vi "Grover Search.vi"   [LabVIEW 2020]
uses:
  QuSim/QuVI_Wire (initial).vi
  QuSim/QuVI_Wire (added).vi
  Gates/Polymorphs/Pauli-X_s.vi
  Gates/Polymorphs/vAControl_e.vi
  Gates/Polymorphs/vAControl_m.vi
  Gates/Polymorphs/Pauli-Z_t.vi
  Gates/Polymorphs/vControl_e.vi
  Gates/Polymorphs/vControl_m.vi
  Analysis/Inspect VIs/Probability Bar.vi
  QuSim/QuWire/QuWire.lvclass
panel:
  # "Grover Search Example"
  # "*Open the block diagram for the circuit view (Ctrl+E)"
  # "Performs Grover's Search algorithm to find a marked item in a 4-qubit space (N=16).\n\nThis VI demonstrates amplitude amplification. It uses a 'For Loop' to iterate the Oracle and Diffusion operators approx. 3 times (optimal for N=16). A 'Case Structure' inside allows you to dynamically select which state (e.g., |1010>) is marked by the Oracle. Watch the probability of the target state rise to >96%."
types:
  T1 = enum16{"0000", "0001", "0010", "0011", "0100", "0101", "0110", "0111", "1000", "1001", "1010", "1011", "1100", "1101", "1110", "1111"}
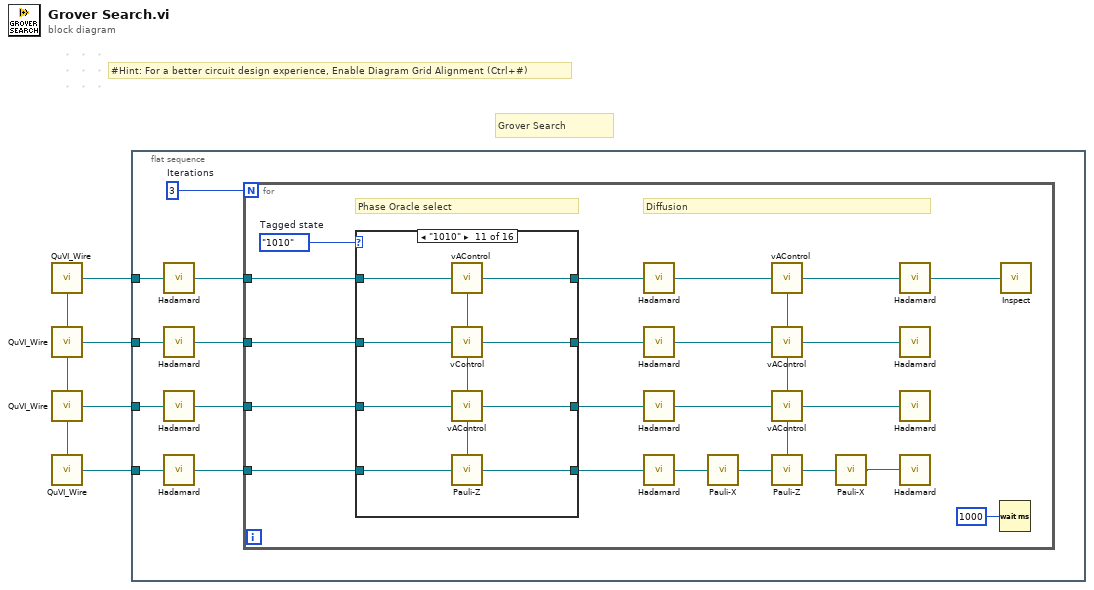
[diagram p0: block diagram]
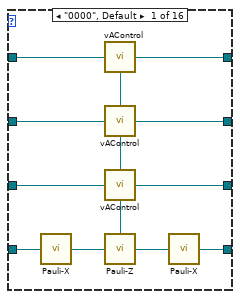
[diagram p2: hidden frame]
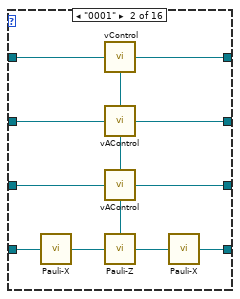
[diagram p3: hidden frame]
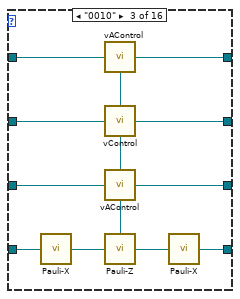
[diagram p4: hidden frame]
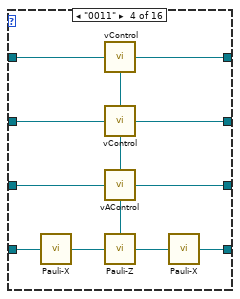
[diagram p5: hidden frame]
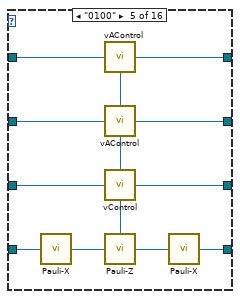
[diagram p6: hidden frame]
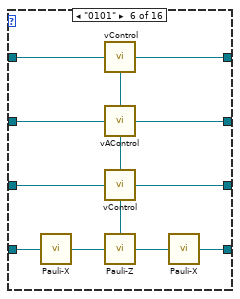
[diagram p7: hidden frame]
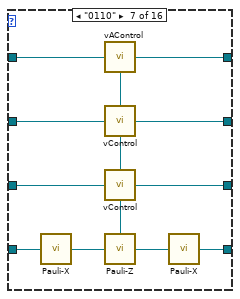
[diagram p8: hidden frame]
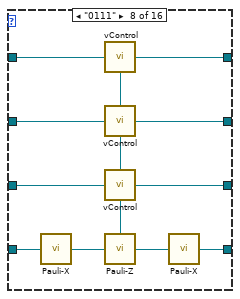
[diagram p9: hidden frame]
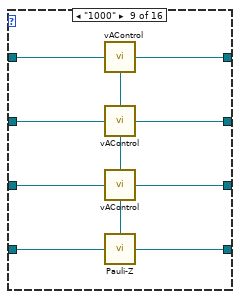
[diagram p10: hidden frame]
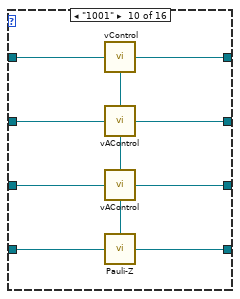
[diagram p11: hidden frame]
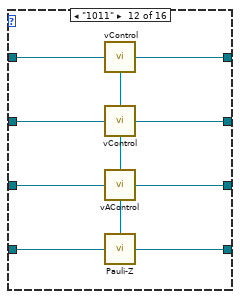
[diagram p12: hidden frame]
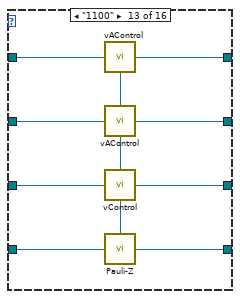
[diagram p13: hidden frame]
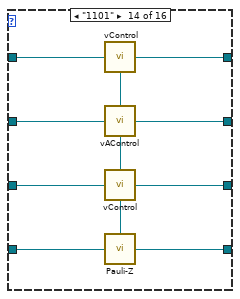
[diagram p14: hidden frame]
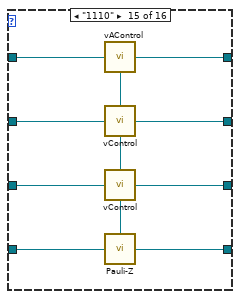
[diagram p15: hidden frame]
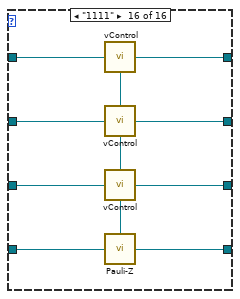
[diagram p16: hidden frame]
diagram:
  # "#Hint: For a better circuit design experience, Enable Diagram Grid Alignment (Ctrl+#)"
  # "Grover Search"
  n1 = call-poly "QuVI_Wire.vi"() -> ("QuWire out"=w5:refnum<class "QuWire.lvclass">, "Stack out"=w7:refnum<class "QuSim.lvclass">)  [unwired: 14 in]
  n2 = call-poly "QuVI_Wire.vi"("Stack in"=w7) -> ("QuWire out"=w6:refnum<class "QuWire.lvclass">, "Stack out"=w3:refnum<class "QuSim.lvclass">)  [unwired: 13 in]
  n3 = call-poly "QuVI_Wire.vi"("Stack in"=w3) -> ("QuWire out"=w4:refnum<class "QuWire.lvclass">, "Stack out"=w1:refnum<class "QuSim.lvclass">)  [unwired: 13 in]
  n4 = call-poly "QuVI_Wire.vi"("Stack in"=w1) -> ("QuWire out"=w2:refnum<class "QuWire.lvclass">)  [unwired: 13 in, 1 out]
  n5 = flat-sequence {
    tunnel: w6 -> [w15]
    tunnel: w5 -> [w16]
    tunnel: w4 -> [w14]
    tunnel: w2 -> [w13]
    frame #0 {
      w12 = 3  # Iterations
      n6 = call "Hadamard.vi"("QuWire in"=w16) -> ("QuWire out"=w9:refnum<class "QuWire.lvclass">)  [unwired: 14 in]
      n7 = call "Hadamard.vi"("QuWire in"=w15) -> ("QuWire out"=w10:refnum<class "QuWire.lvclass">)  [unwired: 14 in]
      n8 = call "Hadamard.vi"("QuWire in"=w14) -> ("QuWire out"=w11:refnum<class "QuWire.lvclass">)  [unwired: 14 in]
      n9 = call "Hadamard.vi"("QuWire in"=w13) -> ("QuWire out"=w8:refnum<class "QuWire.lvclass">)  [unwired: 14 in]
      n10 = for {
        N: w12 -> [_]
        tunnel: w9 -> [w38]
        tunnel: w10 -> [w39]
        tunnel: w11 -> [w40]
        tunnel: w8 -> [w37]
        w19 = T1."1010"  # Tagged state
        # "Phase Oracle select"
        # "Diffusion"
        n11 = case shown="\"1010\"" w19 {
          tunnel: w40 -> [w43 w59 w73 w88 w95 w118 w122 w144 w149 w159 w171 w181 w199 w210 w221 w232]
          tunnel: w39 -> [w53 w66 w68 w82 w105 w117 w125 w134 w155 w166 w172 w182 w198 w209 w216 w224]
          tunnel: w38 -> [w47 w55 w75 w84 w99 w116 w127 w143 w150 w165 w174 w188 w190 w208 w212 w231]
          tunnel: w37 -> [w50 w63 w78 w91 w102 w108 w130 w138 w152 w160 w176 w185 w192 w200 w217 w226]
          tunnel: [w46 w56 w74 w85 w98 w112 w126 w141 w151 w163 w175 w187 w191 w204 w213 w229] -> w36
          tunnel: [w52 w65 w69 w81 w104 w111 w124 w132 w154 w162 w173 w184 w195 w203 w215 w223] -> w35
          tunnel: [w42 w58 w72 w87 w96 w110 w123 w140 w148 w157 w170 w180 w194 w202 w219 w228] -> w34
          tunnel: [w48 w61 w76 w89 w100 w106 w128 w136 w153 w161 w177 w186 w193 w201 w218 w227] -> w33
          frame "0000", Default {
            # "Oracel for 0000 state"
            n12 = call-poly "Pauli-X.vi"("QuWire in"=w50) -> ("QuWire out"=w49:refnum<class "QuWire.lvclass">)  [unwired: 14 in]
            n13 = call-poly "vAControl.vi"("QuWire in"=w47) -> ("QuWire out"=w46:refnum<class "QuWire.lvclass">, "v Ctrl out"=w44:refnum<class "CtrlLine.lvclass">)  [unwired: 13 in]
            n14 = call-poly "vAControl.vi"("v Ctrl in"=w44, "QuWire in"=w53) -> ("QuWire out"=w52:refnum<class "QuWire.lvclass">, "v Ctrl out"=w45:refnum<class "CtrlLine.lvclass">)  [unwired: 12 in]
            n15 = call-poly "vAControl.vi"("v Ctrl in"=w45, "QuWire in"=w43) -> ("QuWire out"=w42:refnum<class "QuWire.lvclass">, "v Ctrl out"=w41:refnum<class "CtrlLine.lvclass">)  [unwired: 12 in]
            n16 = call-poly "Pauli-Z.vi"("v Ctrl  in"=w41, "QuWire in"=w49) -> ("QuWire out"=w51:refnum<class "QuWire.lvclass">)  [unwired: 13 in]
            n17 = call-poly "Pauli-X.vi"("QuWire in"=w51) -> ("QuWire out"=w48:refnum<class "QuWire.lvclass">)  [unwired: 14 in]
          }
          frame "0001" {
            # "Oracel for 0001 state"
            n18 = call-poly "Pauli-X.vi"("QuWire in"=w63) -> ("QuWire out"=w62:refnum<class "QuWire.lvclass">)  [unwired: 14 in]
            n19 = call-poly "vControl.vi"("QuWire in"=w55) -> ("QuWire out"=w56:refnum<class "QuWire.lvclass">, "v Ctrl out"=w54:refnum<class "CtrlLine.lvclass">)  [unwired: 13 in]
            n20 = call-poly "vAControl.vi"("v Ctrl in"=w54, "QuWire in"=w66) -> ("QuWire out"=w65:refnum<class "QuWire.lvclass">, "v Ctrl out"=w60:refnum<class "CtrlLine.lvclass">)  [unwired: 12 in]
            n21 = call-poly "vAControl.vi"("v Ctrl in"=w60, "QuWire in"=w59) -> ("QuWire out"=w58:refnum<class "QuWire.lvclass">, "v Ctrl out"=w57:refnum<class "CtrlLine.lvclass">)  [unwired: 12 in]
            n22 = call-poly "Pauli-Z.vi"("v Ctrl  in"=w57, "QuWire in"=w62) -> ("QuWire out"=w64:refnum<class "QuWire.lvclass">)  [unwired: 13 in]
            n23 = call-poly "Pauli-X.vi"("QuWire in"=w64) -> ("QuWire out"=w61:refnum<class "QuWire.lvclass">)  [unwired: 14 in]
          }
          frame "0010" {
            # "Oracel for 0010 state"
            n24 = call-poly "Pauli-X.vi"("QuWire in"=w78) -> ("QuWire out"=w77:refnum<class "QuWire.lvclass">)  [unwired: 14 in]
            n25 = call-poly "vAControl.vi"("QuWire in"=w75) -> ("QuWire out"=w74:refnum<class "QuWire.lvclass">, "v Ctrl out"=w70:refnum<class "CtrlLine.lvclass">)  [unwired: 13 in]
            n26 = call-poly "vControl.vi"("v Ctrl in"=w70, "QuWire in"=w68) -> ("QuWire out"=w69:refnum<class "QuWire.lvclass">, "v Ctrl out"=w67:refnum<class "CtrlLine.lvclass">)  [unwired: 12 in]
            n27 = call-poly "vAControl.vi"("v Ctrl in"=w67, "QuWire in"=w73) -> ("QuWire out"=w72:refnum<class "QuWire.lvclass">, "v Ctrl out"=w71:refnum<class "CtrlLine.lvclass">)  [unwired: 12 in]
            n28 = call-poly "Pauli-Z.vi"("v Ctrl  in"=w71, "QuWire in"=w77) -> ("QuWire out"=w79:refnum<class "QuWire.lvclass">)  [unwired: 13 in]
            n29 = call-poly "Pauli-X.vi"("QuWire in"=w79) -> ("QuWire out"=w76:refnum<class "QuWire.lvclass">)  [unwired: 14 in]
          }
          frame "0011" {
            # "Oracel for 0011 state"
            n30 = call-poly "Pauli-X.vi"("QuWire in"=w91) -> ("QuWire out"=w90:refnum<class "QuWire.lvclass">)  [unwired: 14 in]
            n31 = call-poly "vControl.vi"("QuWire in"=w84) -> ("QuWire out"=w85:refnum<class "QuWire.lvclass">, "v Ctrl out"=w83:refnum<class "CtrlLine.lvclass">)  [unwired: 13 in]
            n32 = call-poly "vControl.vi"("v Ctrl in"=w83, "QuWire in"=w82) -> ("QuWire out"=w81:refnum<class "QuWire.lvclass">, "v Ctrl out"=w80:refnum<class "CtrlLine.lvclass">)  [unwired: 12 in]
            n33 = call-poly "vAControl.vi"("v Ctrl in"=w80, "QuWire in"=w88) -> ("QuWire out"=w87:refnum<class "QuWire.lvclass">, "v Ctrl out"=w86:refnum<class "CtrlLine.lvclass">)  [unwired: 12 in]
            n34 = call-poly "Pauli-Z.vi"("v Ctrl  in"=w86, "QuWire in"=w90) -> ("QuWire out"=w92:refnum<class "QuWire.lvclass">)  [unwired: 13 in]
            n35 = call-poly "Pauli-X.vi"("QuWire in"=w92) -> ("QuWire out"=w89:refnum<class "QuWire.lvclass">)  [unwired: 14 in]
          }
          frame "0100" {
            # "Oracel for 0100 state"
            n36 = call-poly "Pauli-X.vi"("QuWire in"=w102) -> ("QuWire out"=w101:refnum<class "QuWire.lvclass">)  [unwired: 14 in]
            n37 = call-poly "vAControl.vi"("QuWire in"=w99) -> ("QuWire out"=w98:refnum<class "QuWire.lvclass">, "v Ctrl out"=w97:refnum<class "CtrlLine.lvclass">)  [unwired: 13 in]
            n38 = call-poly "vAControl.vi"("v Ctrl in"=w97, "QuWire in"=w105) -> ("QuWire out"=w104:refnum<class "QuWire.lvclass">, "v Ctrl out"=w93:refnum<class "CtrlLine.lvclass">)  [unwired: 12 in]
            n39 = call-poly "vControl.vi"("v Ctrl in"=w93, "QuWire in"=w95) -> ("QuWire out"=w96:refnum<class "QuWire.lvclass">, "v Ctrl out"=w94:refnum<class "CtrlLine.lvclass">)  [unwired: 12 in]
            n40 = call-poly "Pauli-Z.vi"("v Ctrl  in"=w94, "QuWire in"=w101) -> ("QuWire out"=w103:refnum<class "QuWire.lvclass">)  [unwired: 13 in]
            n41 = call-poly "Pauli-X.vi"("QuWire in"=w103) -> ("QuWire out"=w100:refnum<class "QuWire.lvclass">)  [unwired: 14 in]
          }
          frame "0101" {
            # "Oracel for 0101 state"
            n42 = call-poly "Pauli-X.vi"("QuWire in"=w108) -> ("QuWire out"=w107:refnum<class "QuWire.lvclass">)  [unwired: 14 in]
            n43 = call-poly "vControl.vi"("QuWire in"=w116) -> ("QuWire out"=w112:refnum<class "QuWire.lvclass">, "v Ctrl out"=w115:refnum<class "CtrlLine.lvclass">)  [unwired: 13 in]
            n44 = call-poly "vAControl.vi"("v Ctrl in"=w115, "QuWire in"=w117) -> ("QuWire out"=w111:refnum<class "QuWire.lvclass">, "v Ctrl out"=w114:refnum<class "CtrlLine.lvclass">)  [unwired: 12 in]
            n45 = call-poly "vControl.vi"("v Ctrl in"=w114, "QuWire in"=w118) -> ("QuWire out"=w110:refnum<class "QuWire.lvclass">, "v Ctrl out"=w113:refnum<class "CtrlLine.lvclass">)  [unwired: 12 in]
            n46 = call-poly "Pauli-Z.vi"("v Ctrl  in"=w113, "QuWire in"=w107) -> ("QuWire out"=w109:refnum<class "QuWire.lvclass">)  [unwired: 13 in]
            n47 = call-poly "Pauli-X.vi"("QuWire in"=w109) -> ("QuWire out"=w106:refnum<class "QuWire.lvclass">)  [unwired: 14 in]
          }
          frame "0110" {
            # "Oracel for 0110 state"
            n48 = call-poly "Pauli-X.vi"("QuWire in"=w130) -> ("QuWire out"=w129:refnum<class "QuWire.lvclass">)  [unwired: 14 in]
            n49 = call-poly "vAControl.vi"("QuWire in"=w127) -> ("QuWire out"=w126:refnum<class "QuWire.lvclass">, "v Ctrl out"=w119:refnum<class "CtrlLine.lvclass">)  [unwired: 13 in]
            n50 = call-poly "vControl.vi"("v Ctrl in"=w119, "QuWire in"=w125) -> ("QuWire out"=w124:refnum<class "QuWire.lvclass">, "v Ctrl out"=w120:refnum<class "CtrlLine.lvclass">)  [unwired: 12 in]
            n51 = call-poly "vControl.vi"("v Ctrl in"=w120, "QuWire in"=w122) -> ("QuWire out"=w123:refnum<class "QuWire.lvclass">, "v Ctrl out"=w121:refnum<class "CtrlLine.lvclass">)  [unwired: 12 in]
            n52 = call-poly "Pauli-Z.vi"("v Ctrl  in"=w121, "QuWire in"=w129) -> ("QuWire out"=w131:refnum<class "QuWire.lvclass">)  [unwired: 13 in]
            n53 = call-poly "Pauli-X.vi"("QuWire in"=w131) -> ("QuWire out"=w128:refnum<class "QuWire.lvclass">)  [unwired: 14 in]
          }
          frame "0111" {
            # "Oracel for 0111 state"
            n54 = call-poly "Pauli-X.vi"("QuWire in"=w138) -> ("QuWire out"=w137:refnum<class "QuWire.lvclass">)  [unwired: 14 in]
            n55 = call-poly "vControl.vi"("QuWire in"=w143) -> ("QuWire out"=w141:refnum<class "QuWire.lvclass">, "v Ctrl out"=w135:refnum<class "CtrlLine.lvclass">)  [unwired: 13 in]
            n56 = call-poly "vControl.vi"("v Ctrl in"=w135, "QuWire in"=w134) -> ("QuWire out"=w132:refnum<class "QuWire.lvclass">, "v Ctrl out"=w133:refnum<class "CtrlLine.lvclass">)  [unwired: 12 in]
            n57 = call-poly "vControl.vi"("v Ctrl in"=w133, "QuWire in"=w144) -> ("QuWire out"=w140:refnum<class "QuWire.lvclass">, "v Ctrl out"=w142:refnum<class "CtrlLine.lvclass">)  [unwired: 12 in]
            n58 = call-poly "Pauli-Z.vi"("v Ctrl  in"=w142, "QuWire in"=w137) -> ("QuWire out"=w139:refnum<class "QuWire.lvclass">)  [unwired: 13 in]
            n59 = call-poly "Pauli-X.vi"("QuWire in"=w139) -> ("QuWire out"=w136:refnum<class "QuWire.lvclass">)  [unwired: 14 in]
          }
          frame "1000" {
            # "Oracel for 1 state"
            n60 = call-poly "vAControl.vi"("QuWire in"=w150) -> ("QuWire out"=w151:refnum<class "QuWire.lvclass">, "v Ctrl out"=w145:refnum<class "CtrlLine.lvclass">)  [unwired: 13 in]
            n61 = call-poly "vAControl.vi"("v Ctrl in"=w145, "QuWire in"=w155) -> ("QuWire out"=w154:refnum<class "QuWire.lvclass">, "v Ctrl out"=w146:refnum<class "CtrlLine.lvclass">)  [unwired: 12 in]
            n62 = call-poly "vAControl.vi"("v Ctrl in"=w146, "QuWire in"=w149) -> ("QuWire out"=w148:refnum<class "QuWire.lvclass">, "v Ctrl out"=w147:refnum<class "CtrlLine.lvclass">)  [unwired: 12 in]
            n63 = call-poly "Pauli-Z.vi"("v Ctrl  in"=w147, "QuWire in"=w152) -> ("QuWire out"=w153:refnum<class "QuWire.lvclass">)  [unwired: 13 in]
          }
          frame "1001" {
            # "Oracel for 0101 state"
            n64 = call-poly "vControl.vi"("QuWire in"=w165) -> ("QuWire out"=w163:refnum<class "QuWire.lvclass">, "v Ctrl out"=w164:refnum<class "CtrlLine.lvclass">)  [unwired: 13 in]
            n65 = call-poly "vAControl.vi"("v Ctrl in"=w164, "QuWire in"=w166) -> ("QuWire out"=w162:refnum<class "QuWire.lvclass">, "v Ctrl out"=w158:refnum<class "CtrlLine.lvclass">)  [unwired: 12 in]
            n66 = call-poly "vAControl.vi"("v Ctrl in"=w158, "QuWire in"=w159) -> ("QuWire out"=w157:refnum<class "QuWire.lvclass">, "v Ctrl out"=w156:refnum<class "CtrlLine.lvclass">)  [unwired: 12 in]
            n67 = call-poly "Pauli-Z.vi"("v Ctrl  in"=w156, "QuWire in"=w160) -> ("QuWire out"=w161:refnum<class "QuWire.lvclass">)  [unwired: 13 in]
          }
          frame "1010" {
            # "Oracel for 0101 state"
            n68 = call-poly "vAControl.vi"("QuWire in"=w174) -> ("QuWire out"=w175:refnum<class "QuWire.lvclass">, "v Ctrl out"=w167:refnum<class "CtrlLine.lvclass">)  [unwired: 13 in]
            n69 = call-poly "vControl.vi"("v Ctrl in"=w167, "QuWire in"=w172) -> ("QuWire out"=w173:refnum<class "QuWire.lvclass">, "v Ctrl out"=w168:refnum<class "CtrlLine.lvclass">)  [unwired: 12 in]
            n70 = call-poly "vAControl.vi"("v Ctrl in"=w168, "QuWire in"=w171) -> ("QuWire out"=w170:refnum<class "QuWire.lvclass">, "v Ctrl out"=w169:refnum<class "CtrlLine.lvclass">)  [unwired: 12 in]
            n71 = call-poly "Pauli-Z.vi"("v Ctrl  in"=w169, "QuWire in"=w176) -> ("QuWire out"=w177:refnum<class "QuWire.lvclass">)  [unwired: 13 in]
          }
          frame "1011" {
            # "Oracel for 0101 state"
            n72 = call-poly "vControl.vi"("QuWire in"=w188) -> ("QuWire out"=w187:refnum<class "QuWire.lvclass">, "v Ctrl out"=w183:refnum<class "CtrlLine.lvclass">)  [unwired: 13 in]
            n73 = call-poly "vControl.vi"("v Ctrl in"=w183, "QuWire in"=w182) -> ("QuWire out"=w184:refnum<class "QuWire.lvclass">, "v Ctrl out"=w178:refnum<class "CtrlLine.lvclass">)  [unwired: 12 in]
            n74 = call-poly "vAControl.vi"("v Ctrl in"=w178, "QuWire in"=w181) -> ("QuWire out"=w180:refnum<class "QuWire.lvclass">, "v Ctrl out"=w179:refnum<class "CtrlLine.lvclass">)  [unwired: 12 in]
            n75 = call-poly "Pauli-Z.vi"("v Ctrl  in"=w179, "QuWire in"=w185) -> ("QuWire out"=w186:refnum<class "QuWire.lvclass">)  [unwired: 13 in]
          }
          frame "1100" {
            # "Oracel for 0101 state"
            n76 = call-poly "vAControl.vi"("QuWire in"=w190) -> ("QuWire out"=w191:refnum<class "QuWire.lvclass">, "v Ctrl out"=w189:refnum<class "CtrlLine.lvclass">)  [unwired: 13 in]
            n77 = call-poly "vAControl.vi"("v Ctrl in"=w189, "QuWire in"=w198) -> ("QuWire out"=w195:refnum<class "QuWire.lvclass">, "v Ctrl out"=w197:refnum<class "CtrlLine.lvclass">)  [unwired: 12 in]
            n78 = call-poly "vControl.vi"("v Ctrl in"=w197, "QuWire in"=w199) -> ("QuWire out"=w194:refnum<class "QuWire.lvclass">, "v Ctrl out"=w196:refnum<class "CtrlLine.lvclass">)  [unwired: 12 in]
            n79 = call-poly "Pauli-Z.vi"("v Ctrl  in"=w196, "QuWire in"=w192) -> ("QuWire out"=w193:refnum<class "QuWire.lvclass">)  [unwired: 13 in]
          }
          frame "1101" {
            # "Oracel for 0101 state"
            n80 = call-poly "vControl.vi"("QuWire in"=w208) -> ("QuWire out"=w204:refnum<class "QuWire.lvclass">, "v Ctrl out"=w207:refnum<class "CtrlLine.lvclass">)  [unwired: 13 in]
            n81 = call-poly "vAControl.vi"("v Ctrl in"=w207, "QuWire in"=w209) -> ("QuWire out"=w203:refnum<class "QuWire.lvclass">, "v Ctrl out"=w206:refnum<class "CtrlLine.lvclass">)  [unwired: 12 in]
            n82 = call-poly "vControl.vi"("v Ctrl in"=w206, "QuWire in"=w210) -> ("QuWire out"=w202:refnum<class "QuWire.lvclass">, "v Ctrl out"=w205:refnum<class "CtrlLine.lvclass">)  [unwired: 12 in]
            n83 = call-poly "Pauli-Z.vi"("v Ctrl  in"=w205, "QuWire in"=w200) -> ("QuWire out"=w201:refnum<class "QuWire.lvclass">)  [unwired: 13 in]
          }
          frame "1110" {
            # "Oracel for 0101 state"
            n84 = call-poly "vAControl.vi"("QuWire in"=w212) -> ("QuWire out"=w213:refnum<class "QuWire.lvclass">, "v Ctrl out"=w214:refnum<class "CtrlLine.lvclass">)  [unwired: 13 in]
            n85 = call-poly "vControl.vi"("v Ctrl in"=w214, "QuWire in"=w216) -> ("QuWire out"=w215:refnum<class "QuWire.lvclass">, "v Ctrl out"=w211:refnum<class "CtrlLine.lvclass">)  [unwired: 12 in]
            n86 = call-poly "vControl.vi"("v Ctrl in"=w211, "QuWire in"=w221) -> ("QuWire out"=w219:refnum<class "QuWire.lvclass">, "v Ctrl out"=w220:refnum<class "CtrlLine.lvclass">)  [unwired: 12 in]
            n87 = call-poly "Pauli-Z.vi"("v Ctrl  in"=w220, "QuWire in"=w217) -> ("QuWire out"=w218:refnum<class "QuWire.lvclass">)  [unwired: 13 in]
          }
          frame "1111" {
            # "Oracel for 0101 state"
            n88 = call-poly "vControl.vi"("QuWire in"=w231) -> ("QuWire out"=w229:refnum<class "QuWire.lvclass">, "v Ctrl out"=w225:refnum<class "CtrlLine.lvclass">)  [unwired: 13 in]
            n89 = call-poly "vControl.vi"("v Ctrl in"=w225, "QuWire in"=w224) -> ("QuWire out"=w223:refnum<class "QuWire.lvclass">, "v Ctrl out"=w222:refnum<class "CtrlLine.lvclass">)  [unwired: 12 in]
            n90 = call-poly "vControl.vi"("v Ctrl in"=w222, "QuWire in"=w232) -> ("QuWire out"=w228:refnum<class "QuWire.lvclass">, "v Ctrl out"=w230:refnum<class "CtrlLine.lvclass">)  [unwired: 12 in]
            n91 = call-poly "Pauli-Z.vi"("v Ctrl  in"=w230, "QuWire in"=w226) -> ("QuWire out"=w227:refnum<class "QuWire.lvclass">)  [unwired: 13 in]
          }
        }
        n92 = call "Hadamard.vi"("QuWire in"=w36) -> ("QuWire out"=w32:refnum<class "QuWire.lvclass">)  [unwired: 14 in]
        n93 = call "Hadamard.vi"("QuWire in"=w35) -> ("QuWire out"=w30:refnum<class "QuWire.lvclass">)  [unwired: 14 in]
        n94 = call "Hadamard.vi"("QuWire in"=w34) -> ("QuWire out"=w31:refnum<class "QuWire.lvclass">)  [unwired: 14 in]
        n95 = call "Hadamard.vi"("QuWire in"=w33) -> ("QuWire out"=w24:refnum<class "QuWire.lvclass">)  [unwired: 14 in]
        n96 = call-poly "Pauli-X.vi"("QuWire in"=w24) -> ("QuWire out"=w23:refnum<class "QuWire.lvclass">)  [unwired: 14 in]
        n97 = call-poly "vAControl.vi"("QuWire in"=w32) -> ("QuWire out"=w29:refnum<class "QuWire.lvclass">, "v Ctrl out"=w26:refnum<class "CtrlLine.lvclass">)  [unwired: 13 in]
        n98 = call-poly "vAControl.vi"("v Ctrl in"=w26, "QuWire in"=w30) -> ("QuWire out"=w28:refnum<class "QuWire.lvclass">, "v Ctrl out"=w27:refnum<class "CtrlLine.lvclass">)  [unwired: 12 in]
        n99 = call-poly "vAControl.vi"("v Ctrl in"=w27, "QuWire in"=w31) -> ("QuWire out"=w25:refnum<class "QuWire.lvclass">, "v Ctrl out"=w20:refnum<class "CtrlLine.lvclass">)  [unwired: 12 in]
        n100 = call-poly "Pauli-Z.vi"("v Ctrl  in"=w20, "QuWire in"=w23) -> ("QuWire out"=w22:refnum<class "QuWire.lvclass">)  [unwired: 13 in]
        n101 = call-poly "Pauli-X.vi"("QuWire in"=w22) -> ("QuWire out"=w21:refnum<class "QuWire.lvclass">)  [unwired: 14 in]
        n102 = call "Hadamard.vi"("QuWire in"=w29) -> ("QuWire out"=w17:refnum<class "QuWire.lvclass">)  [unwired: 14 in]
        n103 = call "Hadamard.vi"("QuWire in"=w28) -> ()  [unwired: 14 in, 1 out]
        n104 = call "Hadamard.vi"("QuWire in"=w25) -> ()  [unwired: 14 in, 1 out]
        n105 = call "Hadamard.vi"("QuWire in"=w21) -> ()  [unwired: 14 in, 1 out]
        n106 = Wait (ms)(milliseconds to wait=u32 1000) -> ()  [unwired: 1 out]
        n107 = call-poly "Inspect.vi"("QuWire in"=w17) -> ()  [unwired: 15 in]
      }
    }
  }
